vi "Validate Existing Connections.vi"(8 "error in (no error)":errorcluster, 10 "Missing Identifiers":T1[](array[typedef]), 11 "Routing and Faulting Custom Device Ref in":T2 format="%.0x") -> (0 "error out":errorcluster, 1 "Connection Errors":errorcluster[](array[cluster]), 2 "Invalid Channels":string[](array[string]), 3 "Routing and Faulting Custom Device Ref out":T2 format="%.0x")   [LabVIEW 2017, in "Routing and Faulting Scripting.lvlib"]
uses:
  Routing and Faulting Scripting.lvlib
  <vilib>/NI Veristand/Custom Device API/Custom Device Item Ref.ctl
  Identifier Path Pair.ctl
  <vilib>/NI Veristand/Custom Device API/Custom Device API.lvlib
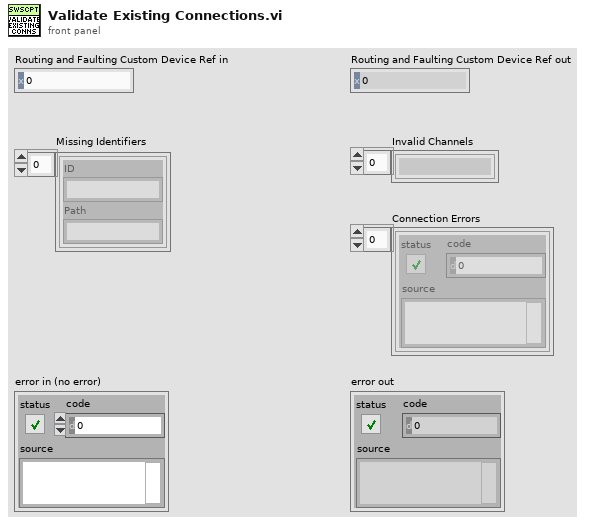
[diagram p1: front panel]
types:
  T1 = typedef "Routing and Faulting Scripting.lvlib/Identifier Path Pair.ctl" = cluster{"ID":string, "Path":string}
  T2 = typedef "Custom Device API.lvlib/Custom Device Item Ref.ctl" = u64
  T3 = typedef "Routing and Faulting Shared.lvlib/Channel States.ctl" = T4[]
  T4 = typedef "Routing and Faulting Shared.lvlib/Routing State.ctl" = cluster{"Name":string, "Description":string, "Value":i32, "Connection List":T5[]}
  T5 = typedef "Routing and Faulting Shared.lvlib/Connection.ctl" = cluster{"Module":string, "Source":string, "Destination":string}
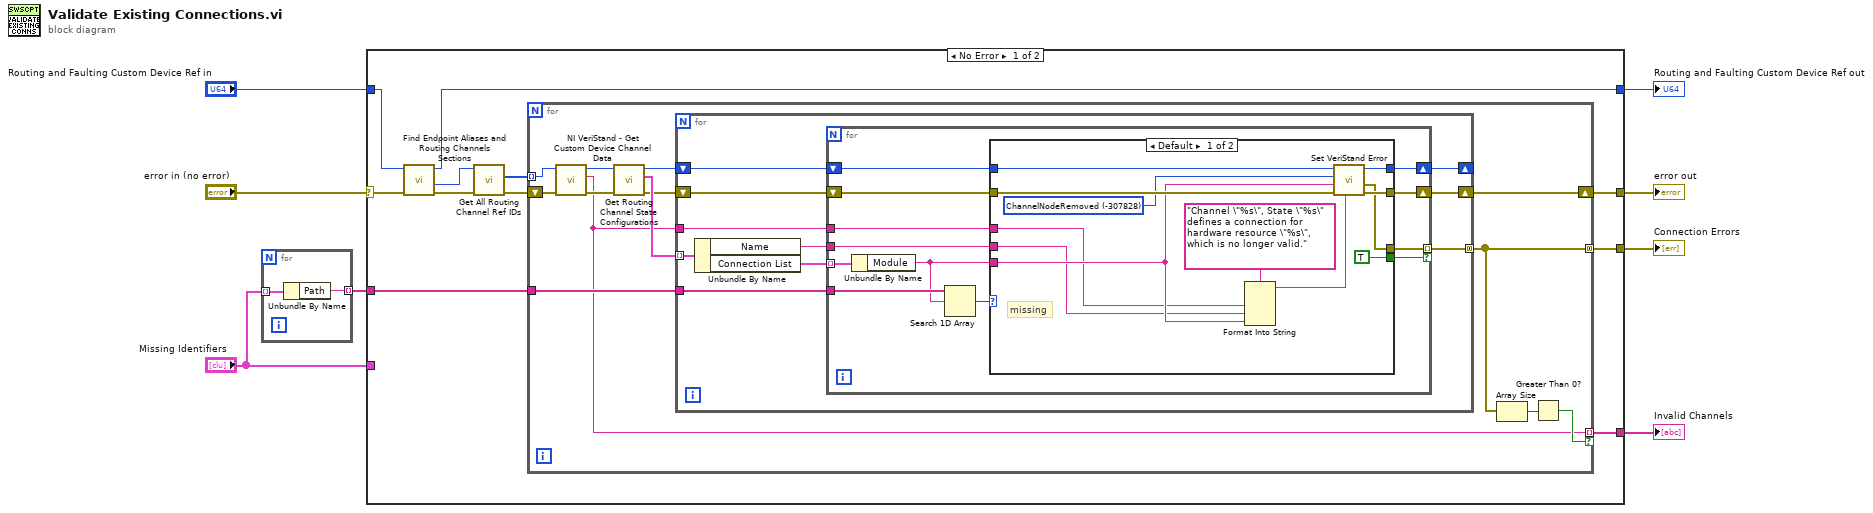
[diagram p0: block diagram]
diagram:
  n1 = for {
    tunnel: "Missing Identifiers" -> [w10] mode=indexing
    tunnel: [w9] -> w3 mode=indexing
    n2 = Unbundle By Name(w10) -> ("Path"=w9:string)
  }
  n3 = case shown="No Error" "error in (no error)" {
    selector: "error in (no error)" -> [w21 w72]
    tunnel: "Routing and Faulting Custom Device Ref in" -> [w20 w71]
    tunnel: [w17 w72] -> w6
    tunnel: [w19 w71] -> w5
    tunnel: "Missing Identifiers" -> [_ _]
    tunnel: w3 -> [w13 _]
    tunnel: [w12 _] -> w2
    tunnel: [w11 _] -> w1
    frame No Error {
      n4 = call "Find Endpoint Aliases and Routing Channels Sections.vi"("error in (no error)"=w21, "Routing and Faulting Custom Device Ref in"=w20) -> ("error out"=w16:errorcluster, "Routing Channels Ref"=w18:T2, "Routing and Faulting Custom Device Ref out"=w19:T2)  [unwired: 6 in, 1 out]
      n5 = call "Get All Routing Channel Ref IDs.vi"("error in (no error)"=w16, "Routing Channels Ref in"=w18) -> ("error out"=w15:errorcluster, "Channel Refs"=w14:T2[])  [unwired: 7 in, 1 out]
      n6 = for {
        tunnel: w14 -> [w28] mode=indexing
        shift-right: [w30] -> w17
        shift-left: w15 -> [w29]
        tunnel: w13 -> [w33]
        tunnel: [w25] -> w12 mode=concatenating
        tunnel: [w22] -> w11 mode=indexing if=w23
        n7 = call <vilib>:"NI VeriStand - Get Custom Device Channel Data.vi"("error in (no error)"=w29, "Channel Ref in"=w28) -> ("error out"=w26:errorcluster, "Channel Name"=w22:string, "Channel Ref out"=w27:T2)  [unwired: 4 in, 3 out]
        n8 = call "Get Routing Channel State Configurations.vi"("error in (no error)"=w26, "Channel Ref in"=w27) -> ("error out"=w32:errorcluster, "State Configurations"=w34:T3, "Channel Ref out"=w31:T2)  [unwired: 7 in]
        n9 = for {
          tunnel: w34 -> [w43] mode=indexing
          tunnel: w33 -> [w42]
          shift-right: [w39] -> w30
          shift-left: w32 -> [w41]
          shift-right: [w38] -> _
          shift-left: w31 -> [w40]
          tunnel: [w36] -> w25 mode=concatenating
          tunnel: w22 -> [w35]
          n10 = Unbundle By Name(w43) -> ("Name"=w37:string, "Connection List"=w44:T5[])
          n11 = for {
            tunnel: w44 -> [w56] mode=indexing
            tunnel: w42 -> [w55]
            shift-right: [w50] -> w39
            shift-left: w41 -> [w53]
            shift-right: [w49] -> w38
            shift-left: w40 -> [w52]
            tunnel: [w48] -> w36 mode=indexing if=w47
            tunnel: w37 -> [w46]
            tunnel: w35 -> [w45]
            n12 = Unbundle By Name(w56) -> ("Module"=w51:string)
            n13 = Search 1D Array(1D array=w55, element=w51) -> (index of element=w54:i32)  [unwired: 1 in]
            n14 = case shown="Default" w54 {
              tunnel: w53 -> [w67 w70]
              tunnel: w52 -> [w66 w69]
              tunnel: w51 -> [w59 _]
              tunnel: [w65 w70] -> w50
              tunnel: [w64 w69] -> w49
              tunnel: [w61 _] -> w48
              tunnel: [TRUE _] -> w47
              tunnel: w46 -> [w58 _]
              tunnel: w45 -> [w57 _]
              frame Default {
                w63 = -307828 items=["Success"=0, "NoProjectOpen"=-307992, "SequenceCompileError"=-307988, "SessionAlreadyDeployed"=-307984, "SessionNotDeployed"=-307982, "SequenceNotFoundInSession"=-307981, "StimulusProfileSessionLocked"=-307980, "EmptyNodeName"=-307930, "NodeAlreadyExistsByName"=-307926, "NumberOfCoefficientsOutOfRange"=-307884, "DownloadFileError"=-307872, "IncorrectLogFileName"=-307871, "LogTriggerConditionSyntaxError"=-307868, "DuplicateLogSessionName"=-307867, "LogSessionNotFound"=-307865, "ChannelLengthMismatch"=-307830, "NodeNotFoundDuringCompile"=-307829, "ChannelNodeRemoved"=-307828, "NotAChannel"=-307825, "NotAWaveform"=-307824, "STIFileError"=-307784, "DependenciesCycle"=-307783, "ChannelNotFoundInLogFile"=-307782, "ChannelGroupNotFoundInLogFile"=-307781, "GatewayNotOnLocalhost"=-307780, "NotEnoughDynamicDataSharingSpace"=-307738, "TargetMissingDataSharingDevice"=-307737, "ChannelMappingsSizeMismatch"=-307728, "DuplicateChannelAliasMappings"=-307711, "NotAnInlineCustomDevice"=-307710, "IncompatibleModel"=-307703, "ModelDimensionMismatch"=-307702, "SLSCChassisLoadFailed"=-307691, "TargetDisabled"=-307689, "MismatchedLengths"=-307687, "TargetInvalid"=-307686, "ParameterNotFound"=-307685, "ServerPortAlreadyInUse"=-307684, "TargetDisconnected"=-307682, "ServiceConfigurationFile"=-307681, "ModelParameterFileParseError"=-307680, "NoActionRequired"=-307677, "InputParameterInvalid"=-307676, "HostRunningDifferentSystemDefinition"=-307671, "ChannelNotScalable"=-307668, "ChannelCannotBeFaulted"=-307666, "ChannelNotWritable"=-307665, "ChannelNotReadable"=-307664, "Timeout"=-307663, "NodeNotFound"=-307662, "SystemDefinitionDeploymentFailure"=-307661, "SystemDefinitionDeploymentTimeout"=-307660, "EmptyPassword"=-307659, "SystemDefinitionAlreadyActive"=-307658, "InvalidConfigurationPassword"=-307657, "NoSystemDefinitionLoaded"=-307656, "ComponentNotAvailable"=-307655, "NotDeployed"=-307654, "InvalidFile"=-307653, "FailedServerConnection"=-307652, "FunctionNotSupported"=-307651, "UnexpectedError"=-307650, "UnmappedAlias"=-307617, "InvalidStreamConditionForDataType"=-307554, "WaveformDataTypeMismatch"=-307553, "InvalidDaqPluginFile"=-307526, "FileVersionUnsupported"=-307525] ("NationalInstruments.VeriStand.ErrorCode")
                # "missing"
                n15 = Format Into String(format string="Channel \"%s\", State \"%s\" defines a connection for hardware resource \"%s\", which is no longer valid.", w57, w58, w59) -> (resulting string=w62:string)  [unwired: 2 in, 1 out]
                n16 = call "Set VeriStand Error.vi"("message"=w62, "error in (no error)"=w67, "key"=w59, "errCode"=w63, "Custom Device Item Ref in"=w66) -> ("error out"=w65:errorcluster, "VeriStand Error out"=w61:errorcluster, "Custom Device Item Ref out"=w64:T2)  [unwired: 4 in]
              }
              frame -1 {
                # "not missing. validate hw connections"
              }
            }
          }
        }
        n17 = Array Size(array=w25) -> (size(s)=w24:i32)
        n18 = Greater Than 0?(x=w24) -> (x > 0?=w23:bool)
      }
    }
    frame Error {
    }
  }
  "Routing and Faulting Custom Device Ref out" <- w5
  "error out" <- w6
  "Connection Errors" <- w2
  "Invalid Channels" <- w1
